vi "Connect.vi"(8 "error in (no error)":errorcluster, 11 "NI-DAQ in":refnum<class "NI-DAQ.lvclass">) -> (0 "error out":errorcluster, 3 "NI-DAQ out":refnum<class "NI-DAQ.lvclass">)   [LabVIEW 2020, in "NI-DAQ.lvclass"]
uses:
  NI-DAQ.lvclass
  NI-DAQ.lvclass/NI-DAQ.ctl
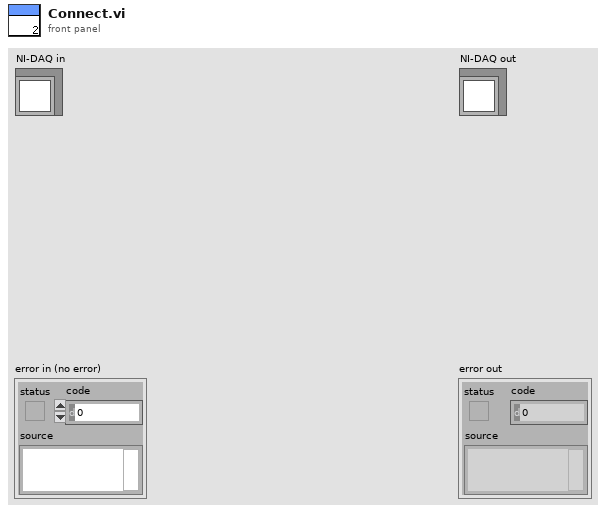
[diagram p1: front panel]
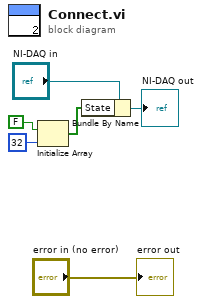
[diagram p0: block diagram]
diagram:
  n1 = Initialize Array(FALSE, 32 ("dimension size")) -> (w3:bool[])
  n2 = Bundle By Name(cluster="NI-DAQ in", "State"=w3) -> (→"NI-DAQ out":refnum<class "NI-DAQ.lvclass">)
  "error out" <- "error in (no error)"
